vi "milan box thingworx.vi"() -> ()   [LabVIEW 2019]
uses:
  Program Files (x86)/National Instruments/LabVIEW 2019/project/EN1Course-master (7)/EN1Course-master/_Subs/ThingWorx/_TW_Subs/TW_XControl.xctl
  <vilib>/httpClient/LabVIEWHTTPClient.lvlib
panel:
  out "decimal integer string":string
  in  "temp":string(xcontrol)
  in  "summary":string(xcontrol)
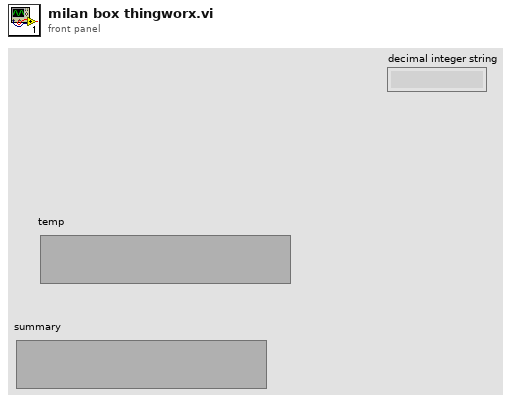
[diagram p1: front panel]
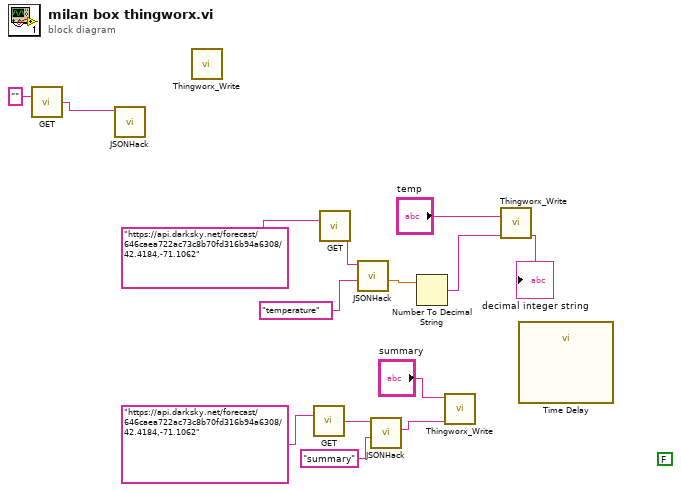
[diagram p0: block diagram]
diagram:
  (unwired) FALSE
  n1 = call <vilib>:"GET.vi"("url"="") -> ("body"=w1:string)  [unwired: 11 in, 3 out]
  n2 = call "JSONHack.vi"("JSON in"=w1) -> ()  [unwired: 7 in, 4 out]
  n3 = call "Thingworx_Write.vi"() -> ()  [unwired: 12 in]
  n4 = call <vilib>:"GET.vi"("url"="https://api.darksky.net/forecast/646caea722ac73c8b70fd316b94a6308/42.4184,-71.1062") -> ("body"=w12:string)  [unwired: 11 in, 3 out]
  n5 = call <vilib>:"GET.vi"("url"="https://api.darksky.net/forecast/646caea722ac73c8b70fd316b94a6308/42.4184,-71.1062") -> ("body"=w9:string)  [unwired: 11 in, 3 out]
  n6 = call "JSONHack.vi"("search name"="temperature", "JSON in"=w9) -> ("Property (num)"=w7:dbl)  [unwired: 6 in, 3 out]
  n7 = call "JSONHack.vi"("search name"="summary", "JSON in"=w12) -> ("Property (str)"=w5:string)  [unwired: 6 in, 3 out]
  n8 = Number To Decimal String(number=w7) -> (decimal integer string=w6:string)  [unwired: 1 in]
  "decimal integer string" <- w6
  n9 = call "Thingworx_Write.vi"("String"=w5, "Thingworx"="summary") -> ()  [unwired: 10 in]
  n10 = call "Thingworx_Write.vi"("String"=w6, "Thingworx"="temp") -> ()  [unwired: 10 in]
  n11 = call "Time Delay"() -> ()  [unwired: 11 in, 1 out]
